vi "blue_square_wave_off_first.vi"(8 "error in":errorcluster, 9 "Iteration":u32, 10 "Device Handle IN":u32, 11 "REACTORS":T1) -> (0 "error out":errorcluster, 1 "Iteration+1":u32, 2 "Device Handle Out":u32, 3 "REACTORS OUT":T1)   [LabVIEW 2013]
uses:
  type_defs/reactor.ctl
  type_defs/reactors.ctl
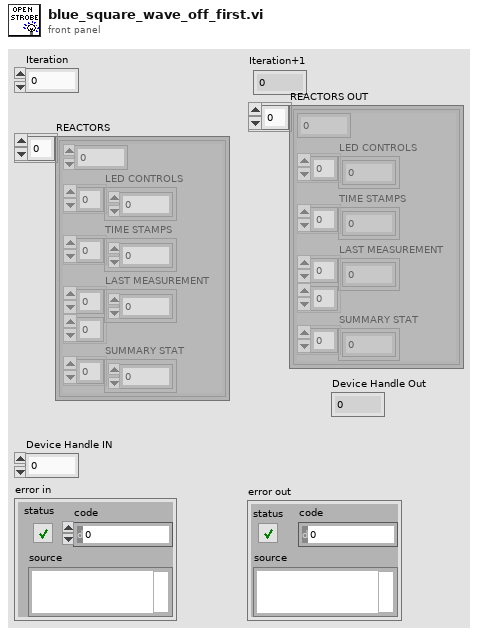
[diagram p1: front panel]
types:
  T1 = typedef "reactors.ctl" = cluster{i32, "LED CONTROLS":dbl[], "TIME STAMPS":dbl[], "LAST MEASUREMENT":T2[][], "SUMMARY STAT":dbl[]}[]
  T2 = typedef "reactor.ctl" = dbl
  T3 = enum16{"Set Mode", "Set Normal Current ", "Set Strobe Parameters", "Set Normal Parameters", "Set Strobe Profile "}
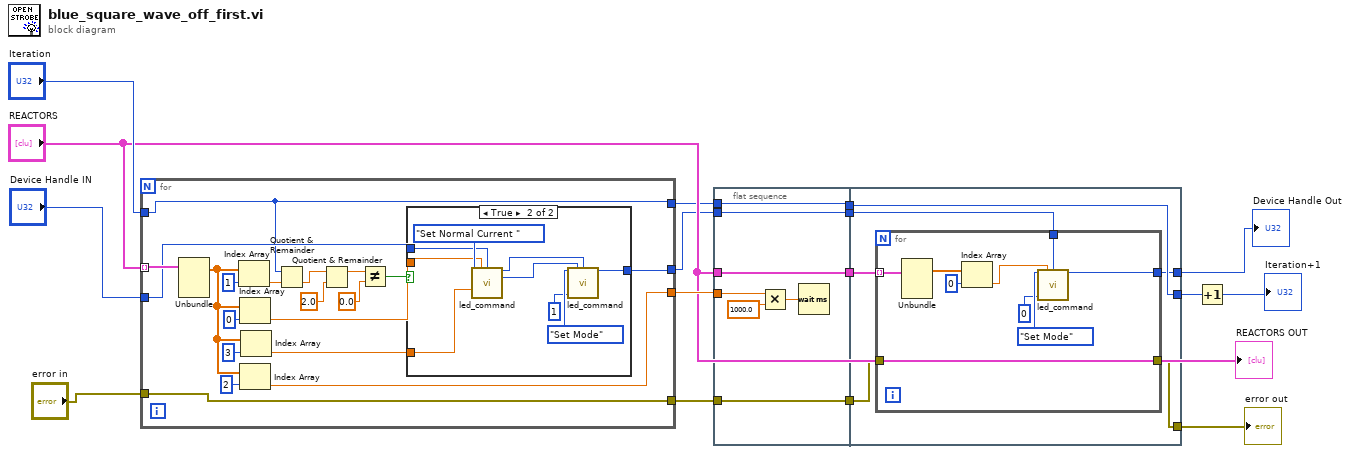
[diagram p0: block diagram]
diagram:
  n1 = for {
    tunnel: "Iteration" -> [w27]
    tunnel: "REACTORS" -> [w35] mode=indexing
    tunnel: "Device Handle IN" -> [w30]
    tunnel: [w29] -> w14
    tunnel: [w28] -> w11
    tunnel: [w27] -> w9
    tunnel: [w26] -> w5
    tunnel: "error in" -> [w26]
    n2 = Unbundle(w35) -> ("LED CONTROLS"=w23:dbl[])  [unwired: 4 out]
    n3 = Index Array(array=w23, index=1) -> (element=w33:dbl)
    n4 = Index Array(array=w23, index=0) -> (element=w31:dbl)
    n5 = Index Array(array=w23, index=2) -> (element=w29:dbl)
    n6 = Index Array(array=w23, index=3) -> (element=w22:dbl)
    n7 = Quotient & Remainder(x=w27, y=w33) -> (floor(x/y)=w20:dbl)  [unwired: 1 out]
    n8 = Quotient & Remainder(x=w20, y=2.0) -> (x-y*floor(x/y)=w19:dbl)  [unwired: 1 out]
    n9 = Not Equal?(x=w19, y=0.0) -> (x != y?=w17:bool)
    n10 = case shown="True" w17 {
      tunnel: w31 -> [_ w38]
      tunnel: w30 -> [w36 w40]
      tunnel: [w36 w43] -> w28
      tunnel: w22 -> [_ w42]
      frame False {
      }
      frame True {
        n11 = call "led_command.vi"("COMMAND"=T3."Set Normal Current ", "Channel"=w38, "Device Handle"=w40, "Iset"=w42) -> ("Device Handle Out"=w39:u32, "Channel Out"=w37:i32)  [unwired: 8 in, 2 out]
        n12 = call "led_command.vi"("COMMAND"=T3."Set Mode", "Channel"=w37, "Device Handle"=w39, "Mode"=u32 1) -> ("Device Handle Out"=w43:u32)  [unwired: 8 in, 3 out]
      }
    }
  }
  n13 = flat-sequence {
    tunnel: "REACTORS" -> [w52]
    tunnel: w14 -> [w51]
    tunnel: [w52] -> w13
    tunnel: w11 -> [w48]
    tunnel: [w48] -> w10
    tunnel: w9 -> [w47]
    tunnel: [w47] -> w8
    tunnel: w5 -> [w46]
    tunnel: [w46] -> w4
    tunnel: w13 -> [w58]
    tunnel: w10 -> [w57]
    tunnel: w8 -> [w56]
    tunnel: [w56] -> w7
    tunnel: w4 -> [w55]
    tunnel: [w54] -> w3
    tunnel: [w53] -> w1
    frame #0 {
      n14 = Multiply(x=w51, y=1000.0) -> (x*y=w50:dbl)
      n15 = Wait (ms)(milliseconds to wait=w50) -> ()  [unwired: 1 out]
    }
    frame #1 {
      n16 = for {
        tunnel: w58 -> [w65] mode=indexing
        tunnel: w57 -> [w62]
        tunnel: w55 -> [w60]
        tunnel: [w60] -> w54
        tunnel: [w59] -> w53
        n17 = Unbundle(w65) -> ("LED CONTROLS"=w66:dbl[])  [unwired: 4 out]
        n18 = Index Array(array=w66, index=0) -> (element=w61:dbl)
        n19 = call "led_command.vi"("COMMAND"=T3."Set Mode", "Channel"=w61, "Device Handle"=w62, "Mode"=u32 0) -> ("Device Handle Out"=w59:u32)  [unwired: 8 in, 3 out]
      }
    }
  }
  n20 = Increment(x=w7) -> (x+1=→"Iteration+1":u32)
  "error out" <- w3
  "REACTORS OUT" <- "REACTORS"
  "Device Handle Out" <- w1
